vi "display_plot.vi"(8 "Y Scale.Name Label.Text":string, 9 "X Scale.Name Label.Text":string, 10 "FileName":string, 11 "Input Data":cluster{"all rows":dbl[], "all rows":dbl[]}(graph)) -> ()   [LabVIEW 2019]
panel:
  out "Output Graph":cluster{"all rows":dbl[], "all rows":dbl[]}(graph)
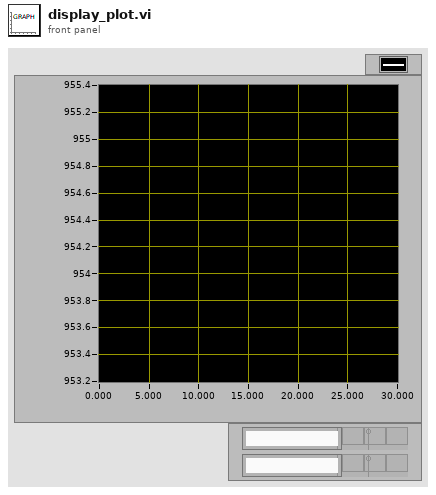
[diagram p1: front panel]
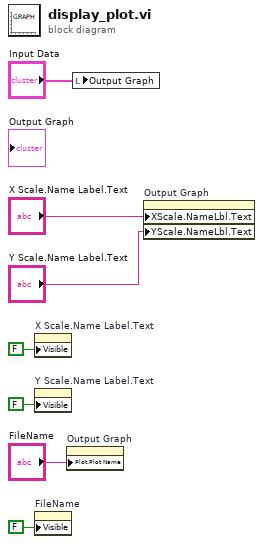
[diagram p0: block diagram]
diagram:
  n1 = property on="X Scale.Name Label.Text" class="Str"("Visible"=FALSE) -> ()  [unwired: 2 in, 2 out]
  n2 = property on="Y Scale.Name Label.Text" class="Str"("Visible"=FALSE) -> ()  [unwired: 2 in, 2 out]
  n3 = property on="FileName" class="Str"("Visible"=FALSE) -> ()  [unwired: 2 in, 2 out]
  n4 = property on="Output Graph" class="XYGraph (strict)"("Plot.Plot Name"="FileName") -> ()  [unwired: 2 in, 2 out]
  n5 = local write "Output Graph"("Input Data") -> ()
  n6 = property on="Output Graph" class="XYGraph (strict)"("XScale.NameLbl.Text"="X Scale.Name Label.Text", "YScale.NameLbl.Text"="Y Scale.Name Label.Text") -> ()  [unwired: 2 in, 2 out]
